vi "Axis ref manager.vi"(5 "Index/size in":u32, 6 "Ref in":refnum<vi>, 7 "Mode":enum16{"Init", "Set", "Get"}(ring)) -> (2 "Ref out":refnum<vi>)   [LabVIEW 2019]
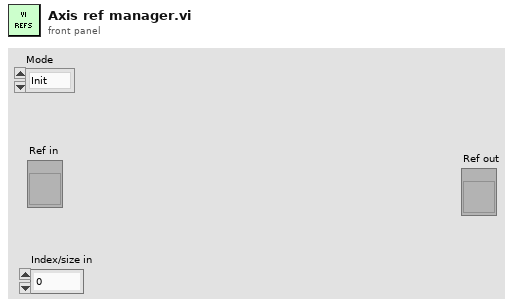
[diagram p1: front panel]
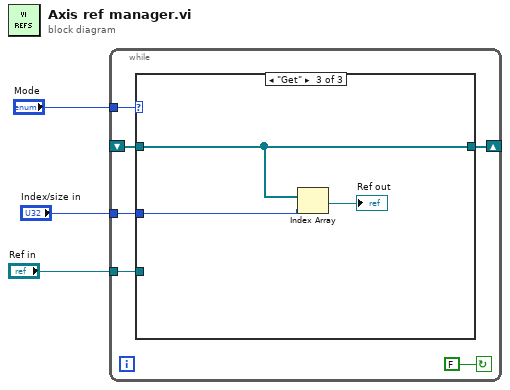
[diagram p0: block diagram]
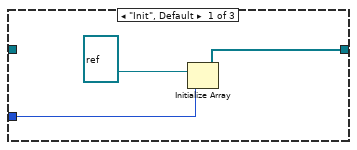
[diagram p2: hidden frame]
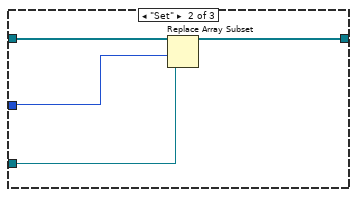
[diagram p3: hidden frame]
diagram:
  n1 = while {
    tunnel: "Mode" -> [w8]
    shift-right: [w6] -> _
    shift-left: _ -> [w5]
    tunnel: "Index/size in" -> [w7]
    tunnel: "Ref in" -> [w4]
    stop <- FALSE continue-if-true
    n2 = case shown="\"Get\"" w8 {
      tunnel: w7 -> [w11 w13 w17]
      tunnel: [w10 w15 w19] -> w6
      tunnel: w5 -> [_ w16 w19]
      tunnel: w4 -> [_ w14 _]
      frame "Init", Default {
        n3 = Initialize Array(refnum<vi> refnum ("This VI"), w11) -> (w10:refnum<vi>[])
      }
      frame "Set" {
        n4 = Replace Array Subset(array=w16, new element=w14, index=w13) -> (w15:refnum<vi>[])
      }
      frame "Get" {
        n5 = Index Array(array=w19, index=w17) -> (element=→"Ref out":refnum<vi>)
      }
    }
  }
